vi "DataLogWrite.vi"() -> ()   [LabVIEW 2023]
uses:
  impl_ControlRecordType_ENUM.ctl
  <vilib>/numeric/Random Number (Range) I64.vi
  <vilib>/Rock Robotics/WPI/ThirdParty/JAS_Junk/TrajLib/Trajectory_Library.lvlib
panel:
  out "string":string
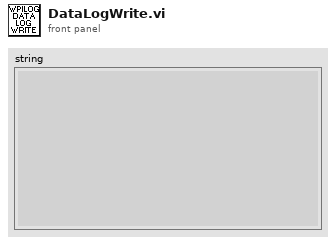
[diagram p1: front panel]
types:
  T1 = enum16{"big-endian, network order", "native, host order", "little-endian"}
  T2 = typedef "impl_ControlRecordType_ENUM.ctl" = enum16{"kControlStart", "kControlFinish", "kControlSetMetadata"}
  T3 = cluster{"entry ID being started/completed/updated":i32, "entry name UTF-8 string data (arbitrary length)":string, "entry type UTF-8 string data (arbitrary length)":string, "entry metadata UTF-8 string data (arbitrary length)":string}
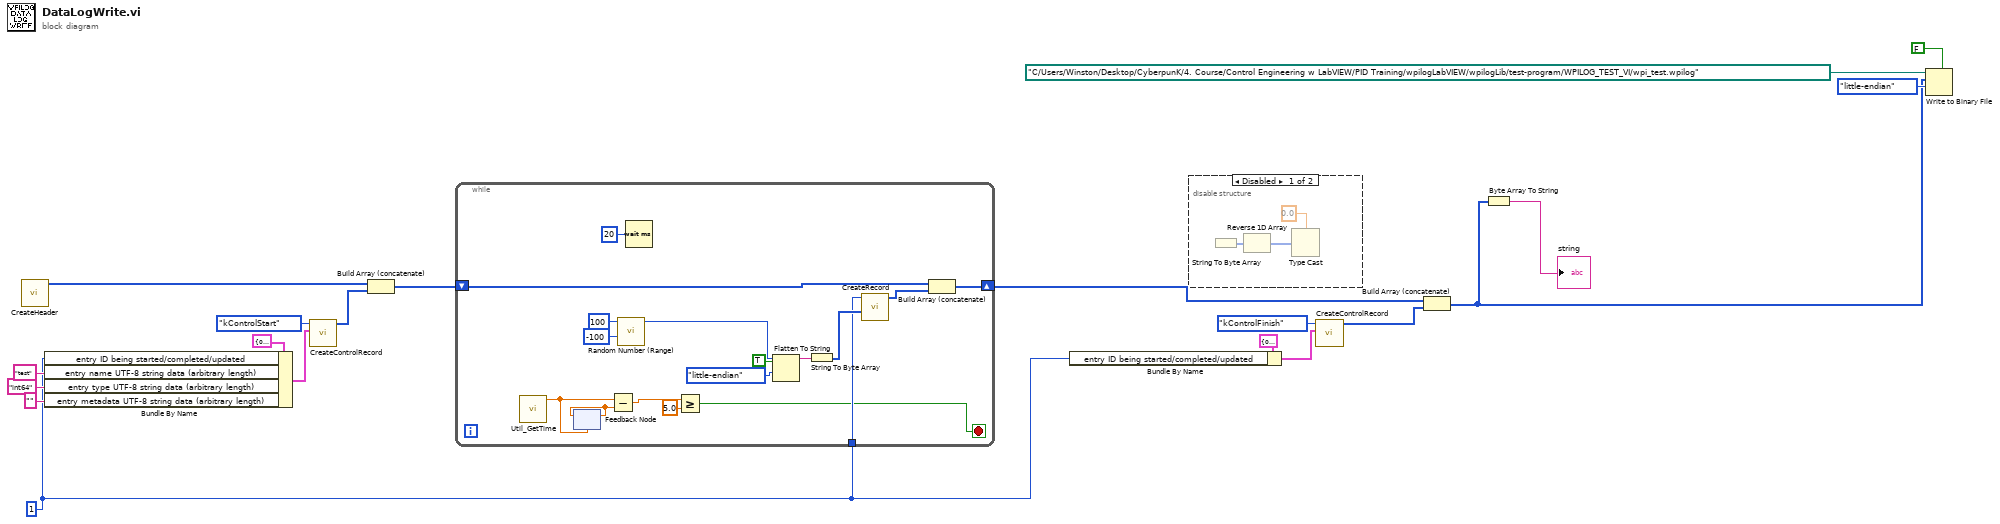
[diagram p0: block diagram]
diagram:
  w1 = 1 ("entry ID being started/completed/updated")
  n1 = call "CreateHeader.vi"() -> ("header"=w16:u8[])  [unwired: 11 in]
  n2 = Bundle By Name(cluster=T3 {"entry ID being started/completed/updated"=0, "entry name UTF-8 string data (arbitrary length)"="", "entry type UTF-8 string data (arbitrary length)"="", "entry metadata UTF-8 string data (arbitrary length)"=""} ("Control Record Payload Data"), "entry ID being started/completed/updated"=w1, "entry name UTF-8 string data (arbitrary length)"="test", "entry type UTF-8 string data (arbitrary length)"="int64", "entry metadata UTF-8 string data (arbitrary length)"="") -> (w18:T3)
  n3 = call "CreateControlRecord.vi"("Control Record Payload Data"=w18, "ControlRecordType"=impl_ControlRecordType_ENUM."kControlStart") -> ("control record"=w17:u8[])  [unwired: 9 in]
  n4 = Build Array (concatenate)(w16, w17) -> (w12:u8[])
  n5 = while {
    tunnel: w1 -> [w30]
    shift-right: [w31] -> w7
    shift-left: w12 -> [w33]
    stop <- w21 stop-if-true
    n6 = call <vilib>:"Util_GetTime.vi"() -> ("FPGA_Time_Seconds"=w23:dbl)  [unwired: 9 in, 2 out]
    n7 = feedback #1(w23) -> (w24:dbl)
    n8 = feedback-in #1(w24) -> ()
    n9 = Subtract(x=w23, y=w24) -> (x-y=w22:dbl)
    n10 = call-poly <vilib>:"Random Number (Range).vi"("lower bound (-100)"=i64 -100, "upper bound (100)"=i64 100) -> ("number"=w27:i64)  [unwired: 9 in]
    n11 = Wait (ms)(milliseconds to wait=u32 20) -> ()  [unwired: 1 out]
    n12 = Greater Or Equal?(x=w22, y=5.0) -> (x >= y?=w21:bool)
    n13 = Flatten To String(anything=w27, prepend array or string size? (T)=TRUE, byte order (0:big-endian, network order)=T1."little-endian") -> (data string=w35:string)  [unwired: 1 in, 2 out]
    n14 = String To Byte Array(string=w35) -> (unsigned byte array=w34:u8[])
    n15 = call "CreateRecord.vi"("payload data (little endian)"=w34, "entry ID"=w30) -> ("record"=w32:u8[])  [unwired: 9 in]
    n16 = Build Array (concatenate)(w33, w32) -> (w31:u8[])
  }
  n17 = Bundle By Name(cluster=T3 {"entry ID being started/completed/updated"=0, "entry name UTF-8 string data (arbitrary length)"="", "entry type UTF-8 string data (arbitrary length)"="", "entry metadata UTF-8 string data (arbitrary length)"=""} ("Control Record Payload Data"), "entry ID being started/completed/updated"=w1) -> (w11:T3)
  n18 = disable-structure shown="Disabled" {
    frame Disabled {
      n19 = String To Byte Array() -> (unsigned byte array=w40:u8[])  [unwired: 1 in]
      n20 = Reverse 1D Array(array=w40) -> (reversed array=w39:u8[])
      n21 = Type Cast(type=0.0, x=w39) -> ()  [unwired: 1 out]
    }
    frame Enabled {
    }
  }
  n22 = call "CreateControlRecord.vi"("Control Record Payload Data"=w11, "ControlRecordType"=impl_ControlRecordType_ENUM."kControlFinish") -> ("control record"=w8:u8[])  [unwired: 9 in]
  n23 = Build Array (concatenate)(w7, w8) -> (w4:u8[])
  n24 = Byte Array To String(unsigned byte array=w4) -> (string=→"string":string)
  n25 = Write to Binary File(file (use dialog)=path "C:/Users/Winston/Desktop/CyberpunK/4. Course/Control Engineering w LabVIEW/PID Training/wpilogLabVIEW/wpilogLib/test-program/WPILOG_TEST_VI/wpi_test.wpilog", data=w4, 5:FALSE ("prepend array or string size? (T)"), 9:T1."little-endian" ("byte order (0:big-endian, network order)")) -> ()  [unwired: 2 in, 3 out]
